vi "Set Configuration File Path.vi"(8 "error in":errorcluster, 10 "configuration file path":path, 11 "custom device ref in":T1 format="%.0x") -> (0 "error out":errorcluster, 3 "custom device ref out":T1 format="%.0x")   [LabVIEW 2020, in "AIM ARINC 664 Scripting.lvlib"]
uses:
  AIM ARINC 664 Scripting.lvlib
  <vilib>/NI VeriStand/Custom Device API/Custom Device Item Ref.ctl
  Constants.vi
  <vilib>/NI VeriStand/Custom Device Tools/Custom Device Utility Library/NI VeriStand - Search for Item by GUID.vi
  <vilib>/NI VeriStand/Custom Device API/Set Item Property (Dependent File).vi
  <vilib>/NI VeriStand/Custom Device Tools/Custom Device Utility Library/Custom Device Utility Library.lvlib
  <vilib>/NI VeriStand/Custom Device API/Custom Device API.lvlib
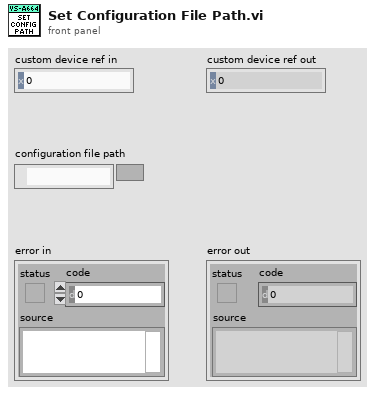
[diagram p1: front panel]
types:
  T1 = typedef "Custom Device API.lvlib/Custom Device Item Ref.ctl" = u64
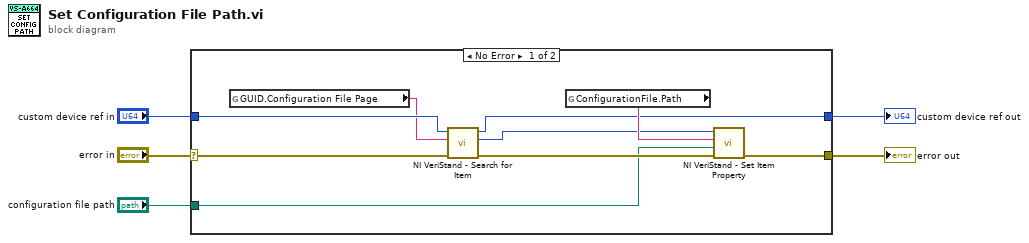
[diagram p0: block diagram]
diagram:
  n1 = case shown="No Error" "error in" {
    selector: "error in" -> [w11 w16]
    tunnel: "custom device ref in" -> [w12 w15]
    tunnel: [w14 w16] -> w4
    tunnel: [w7 w15] -> w3
    tunnel: "configuration file path" -> [w6 _]
    frame No Error {
      n2 = global read "Constants.vi" "GUID.Configuration File Page"() -> (w9:string)
      n3 = call-poly <vilib>:"NI VeriStand - Search for Item.vi"("error in"=w11, "Item GUID"=w9, "Section Ref in"=w12) -> ("error out"=w10:errorcluster, "Item Ref"=w8:T1, "Section Ref out"=w7:T1)  [unwired: 5 in, 1 out]
      n4 = global read "Constants.vi" "ConfigurationFile.Path"() -> (w13:string)
      n5 = call-poly <vilib>:"NI VeriStand - Set Item Property.vi"("error in (no error)"=w10, "Path"=w6, "Property Name"=w13, "Item Ref in"=w8) -> ("error out"=w14:errorcluster)  [unwired: 5 in, 2 out]
    }
    frame Error {
    }
  }
  "error out" <- w4
  "custom device ref out" <- w3
